vi "Fixture.vi"(8 "error in (no error)":errorcluster, 11 "Color":u32) -> (0 "error out":errorcluster, 3 "SceneObject out":refnum<vi>)   [LabVIEW 2026, in "XRay CArm.lvclass"]
uses:
  XRay CArm.lvclass
  <vilib>/picture/3D Picture Control/Object/Create Object (drawable).vi
  <vilib>/picture/3D Picture Control/NI_3D Picture Control.lvlib
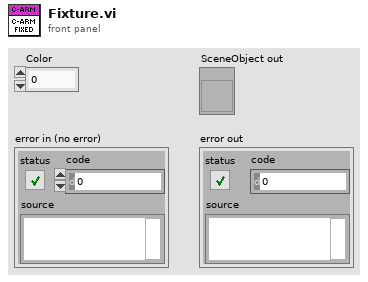
[diagram p1: front panel]
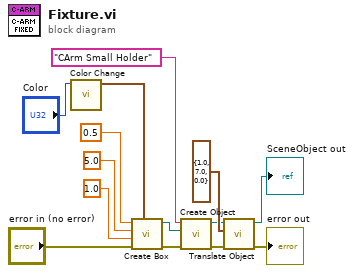
[diagram p0: block diagram]
diagram:
  n1 = call <vilib>:"Color Change.vi"("Color"="Color") -> ("RGBA"=w2:cluster{"R":sgl, "G":sgl, "B":sgl, "A":sgl})  [unwired: 10 in]
  n2 = call <vilib>:"Create Box.vi"("Color"=w2, "error in (no error)"="error in (no error)", "Length Z"=sgl 1.0 ("Box Length Z"), "Length Y"=sgl 5.0 ("Box Length Y"), "Length X"=sgl 0.5 ("Box Length X")) -> ("error out"=w4:errorcluster, "New Box Refnum"=w5:refnum<vi>)  [unwired: 5 in]
  n3 = call-poly <vilib>:"Create Object.vi"("error in (no error)"=w4, "Geometry"=w5, "Name"="CArm Small Holder") -> ("error out"=w11:errorcluster, "Scene:New Object"=w6:refnum<vi>)  [unwired: 7 in]
  n4 = call <vilib>:"Translate Object.vi"("error in (no error)"=w11, "Translation"=cluster{"X":sgl, "Y":sgl, "Z":sgl} {"X"=1.0, "Y"=7.0, "Z"=0.0}, "Scene.Object In"=w6) -> ("error out"=→"error out":errorcluster, "Scene.Object Out"=→"SceneObject out":refnum<vi>)  [unwired: 7 in]
